vi "user32_GetMenu.vi"(8 "错误输入（无错误）":errorcluster, 11 "hWnd":u32) -> (0 "错误输出":errorcluster, 1 "success?":bool, 2 "hMenu":u32, 3 "dup hWnd":u32)   [LabVIEW 2011]
doc: "该函数取得分配给指定窗口的菜单的句柄。"
uses:
  user32.dll
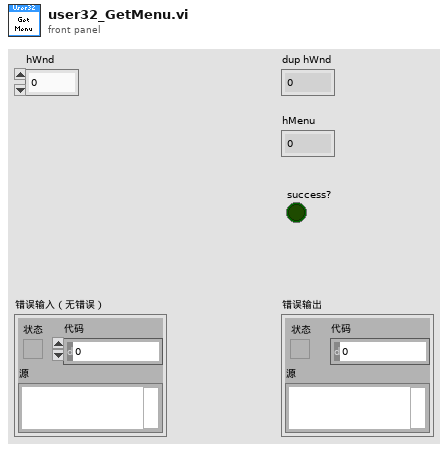
[diagram p1: front panel]
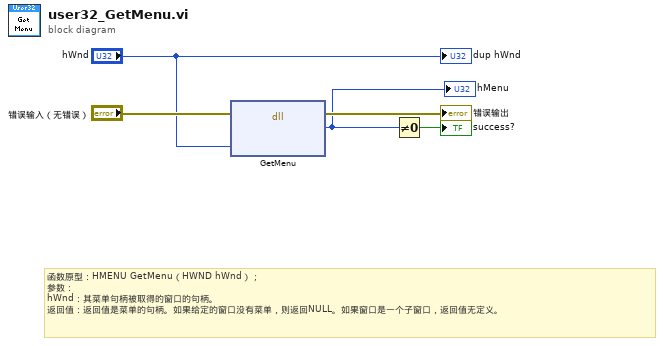
[diagram p0: block diagram]
diagram:
  # "函数原型：HMENU GetMenu（HWND hWnd）；\n参数：\nhWnd：其菜单句柄被取得的窗口的句柄。\n返回值：返回值是菜单的句柄。如果给定的窗口没有菜单，则返回NULL。如果窗口是一个子窗口，返回值无定义。"
  n1 = dll-call lib="user32.dll" fn="GetMenu"(error in="错误输入（无错误）", "hWnd"="hWnd") -> (error out=→"错误输出":errorcluster, "hMenu"=w2:u32)  [unwired: 3 in, 1 out]
  "hMenu" <- w2
  n2 = Not Equal To 0?(x=w2) -> (x != 0?=→"success?":bool)
  "dup hWnd" <- "hWnd"
